vi "Init.vi"(8 "error in (no error)":errorcluster, 11 "Input Name":string) -> (0 "error out":errorcluster, 3 "GetInputSettings out":refnum<class "GetInputSettings.lvclass">)   [LabVIEW 2020, in "obs-websocket.lvlib" / "GetInputSettings.lvclass"]
uses:
  GetInputSettings.lvclass
  GetInputSettings.lvclass/GetInputSettings.ctl
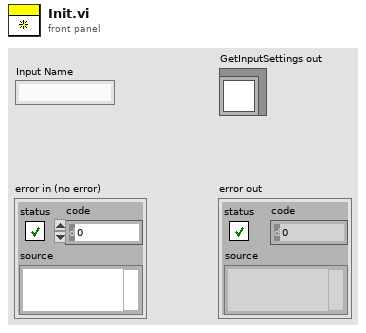
[diagram p1: front panel]
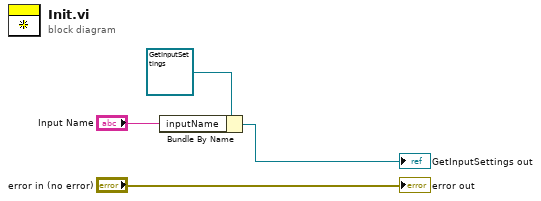
[diagram p0: block diagram]
diagram:
  n1 = Bundle By Name(cluster=refnum<class "GetInputSettings.lvclass"> refnum ("GetInputSettings in"), "inputName"="Input Name") -> (→"GetInputSettings out":refnum<class "GetInputSettings.lvclass">)
  "error out" <- "error in (no error)"
